vi "Update_Caliper_Overlay_dll.vi"(5 "Analysis_Point_Result":T2[](array[typedef]), 7 "CaliperEntry":T3 {"CaliperType" items=["Distance", "Mid Point", "Perpendicular Projection", "Lines Intersection", "Angle from Horizontal", "Angle from Vertical", "Angle Defined by 3 Points", "Angle Defined by 4 Points", "Bissecting Line", "Mid Line", "Center of Mass", "Area", "Line Fit", "Circle Fit", "Ellipse Fit"]}, 10 "OverlayColor":u32(colorbox)=16711680, 11 "DLL Vision_Image":T1) -> (3 "DLL Vision_Image Out":T1)   [LabVIEW 2019]
uses:
  Caliper/Controls/CaliperDataEntry.ctl
  Caliper/Controls/CaliperType.ctl
  Caliper/Controls/SelectionListEntry.ctl
  Caliper/Controls/SelectionListEntryPointType.ctl
  Caliper/Controls/CaliperResult.ctl
  Analysis/Controls/Analysis_Result_To_Caliper.ctl
  <vilib>/vision/Image Controls.llb/IMAQ Image.ctl
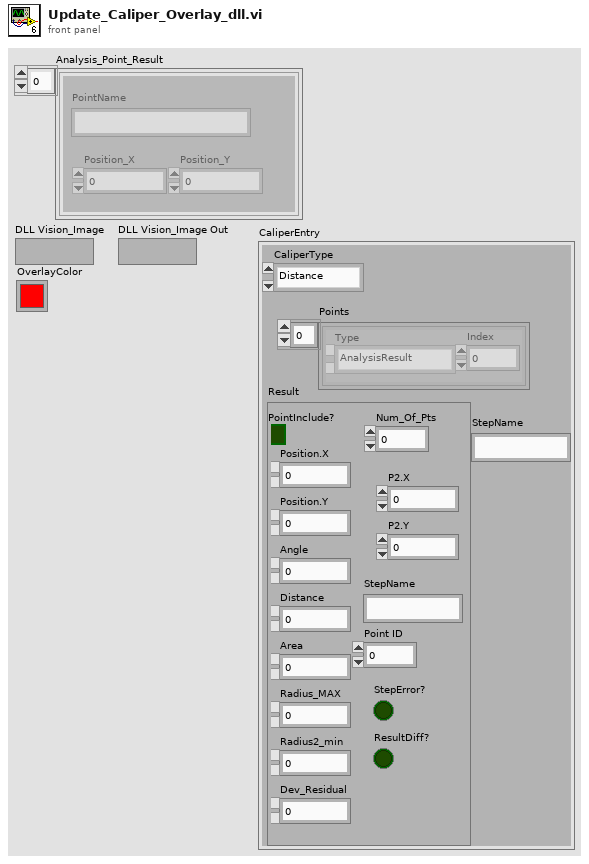
[diagram p1: front panel]
types:
  T1 = typedef "IMAQ Image.ctl" = refnum<image>
  T2 = typedef "Analysis_Result_To_Caliper.ctl" = cluster{"PointName":string, "Position_X":dbl, "Position_Y":dbl}
  T3 = typedef "CaliperDataEntry.ctl" = cluster{"CaliperType":T4, "Points":T5[], "Result":T7, "StepName":string}
  T4 = typedef "CaliperType.ctl" = u32
  T5 = typedef "SelectionListEntry.ctl" = cluster{"Type":T6, "Index":i32}
  T6 = typedef "SelectionListEntryPointType.ctl" = enum16{"AnalysisResult", "CaliperResult"}
  T7 = typedef "CaliperResult.ctl" = cluster{"PointInclude?":bool, "Num_Of_Pts":u8, "Position.X":dbl, "Position.Y":dbl, "Angle":dbl, "Distance":dbl, "Area":dbl, "Radius_MAX":dbl, "Radius2_min":dbl, "Dev_Residual":dbl, "P2.X":dbl, "P2.Y":dbl, "StepName":string, "Point ID":u8, "StepError?":bool, "ResultDiff?":bool}
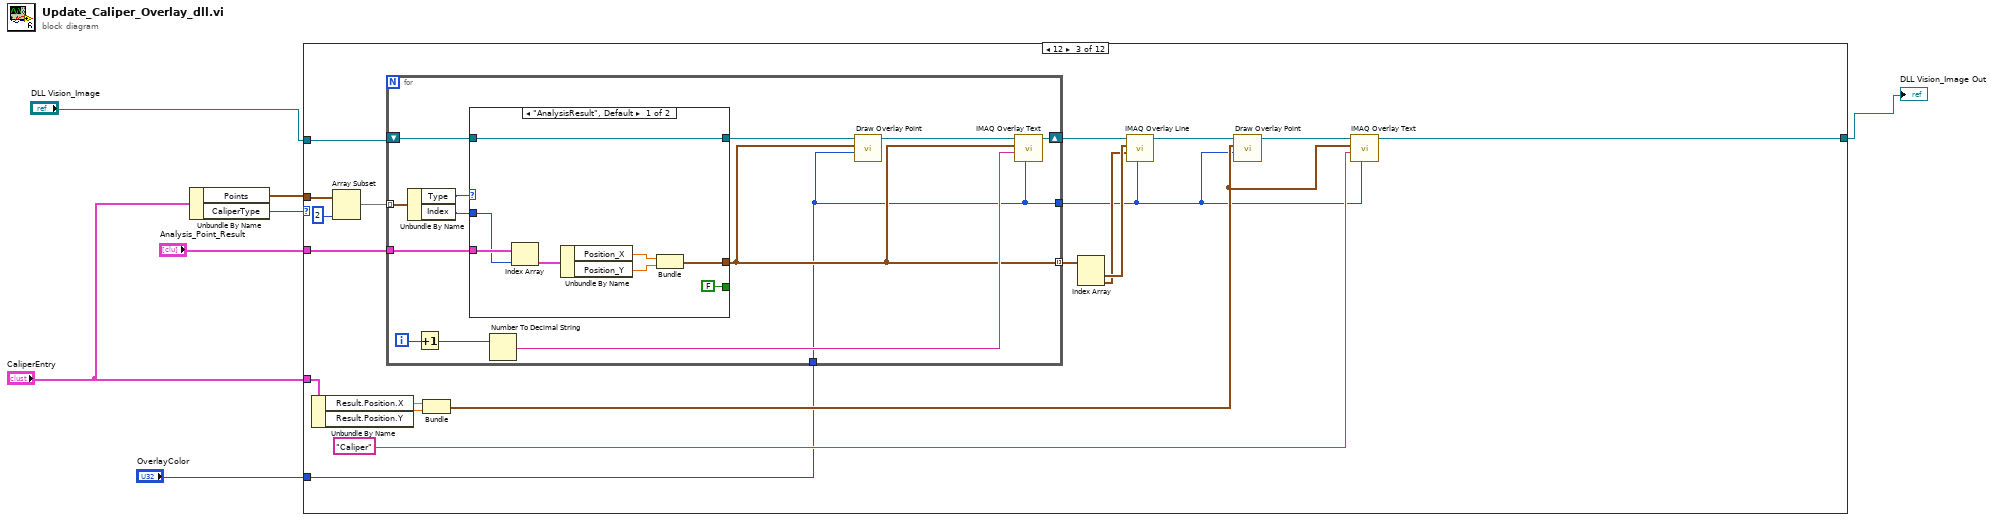
[diagram p0: block diagram]
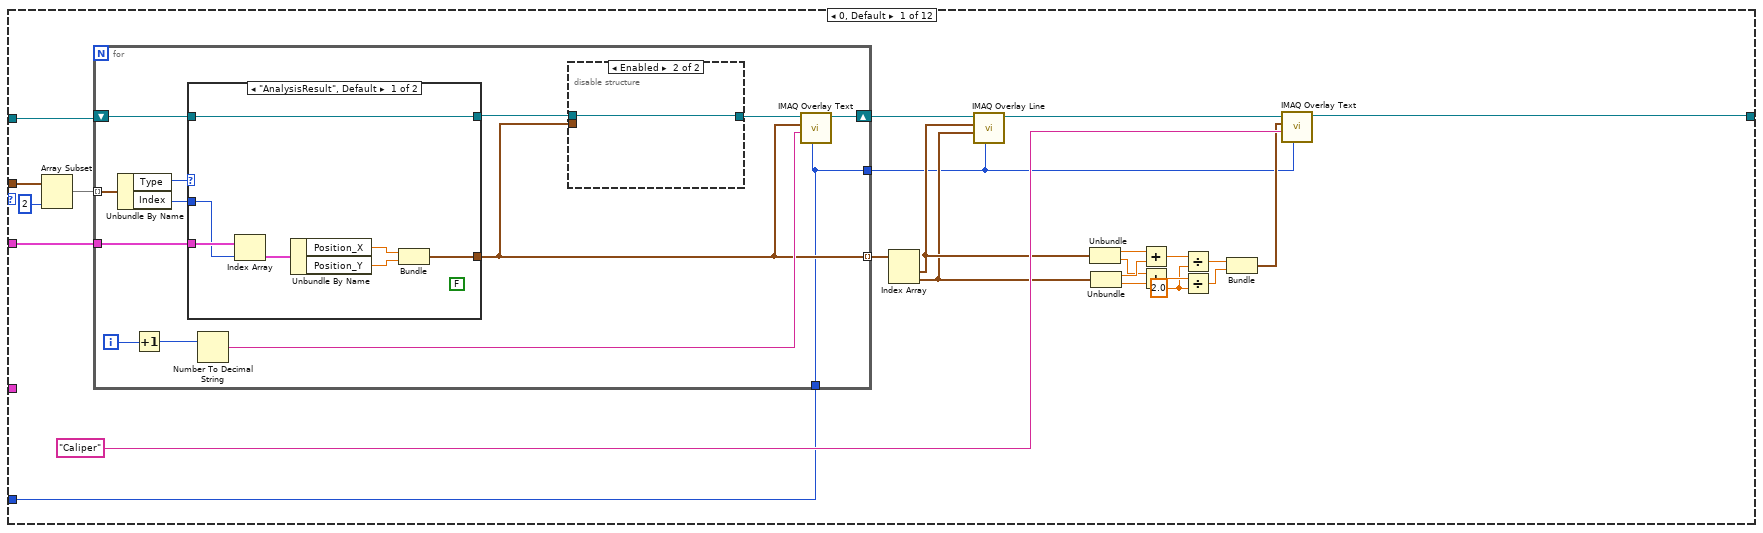
[diagram p2: hidden frame]
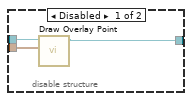
[diagram p3: hidden frame]
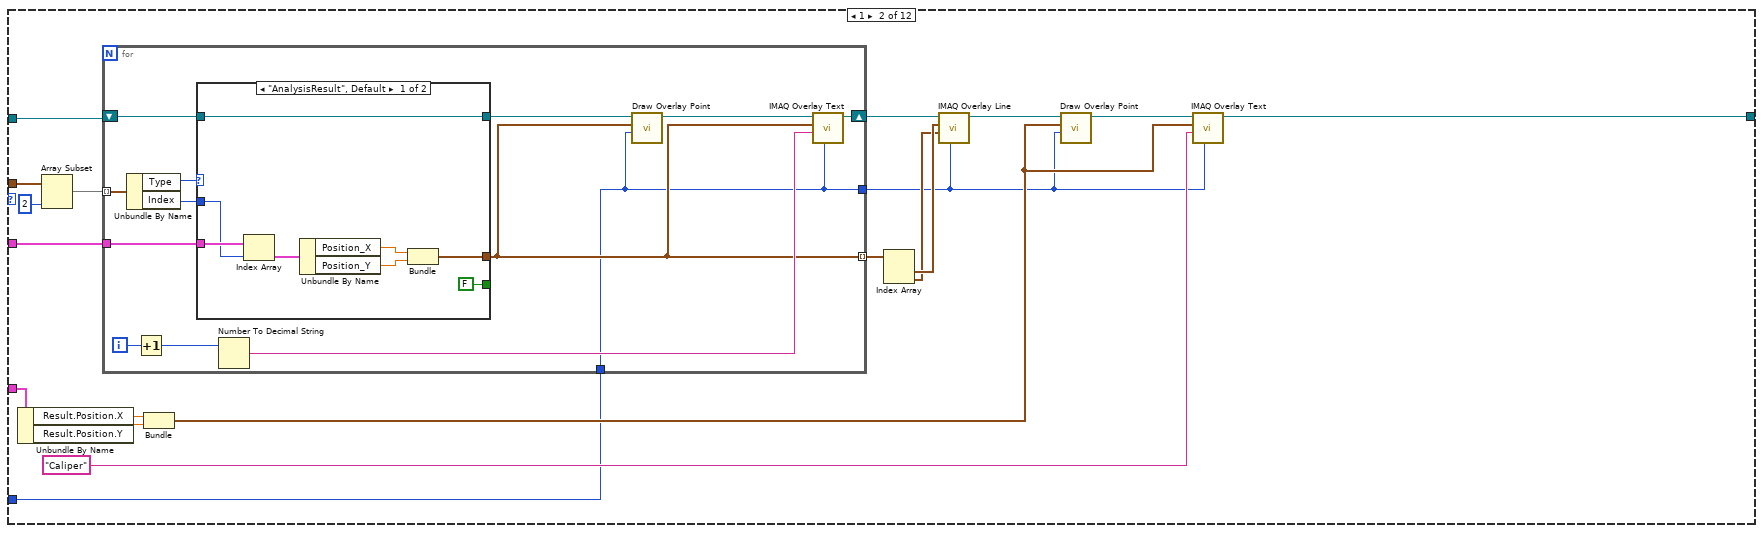
[diagram p5: hidden frame]
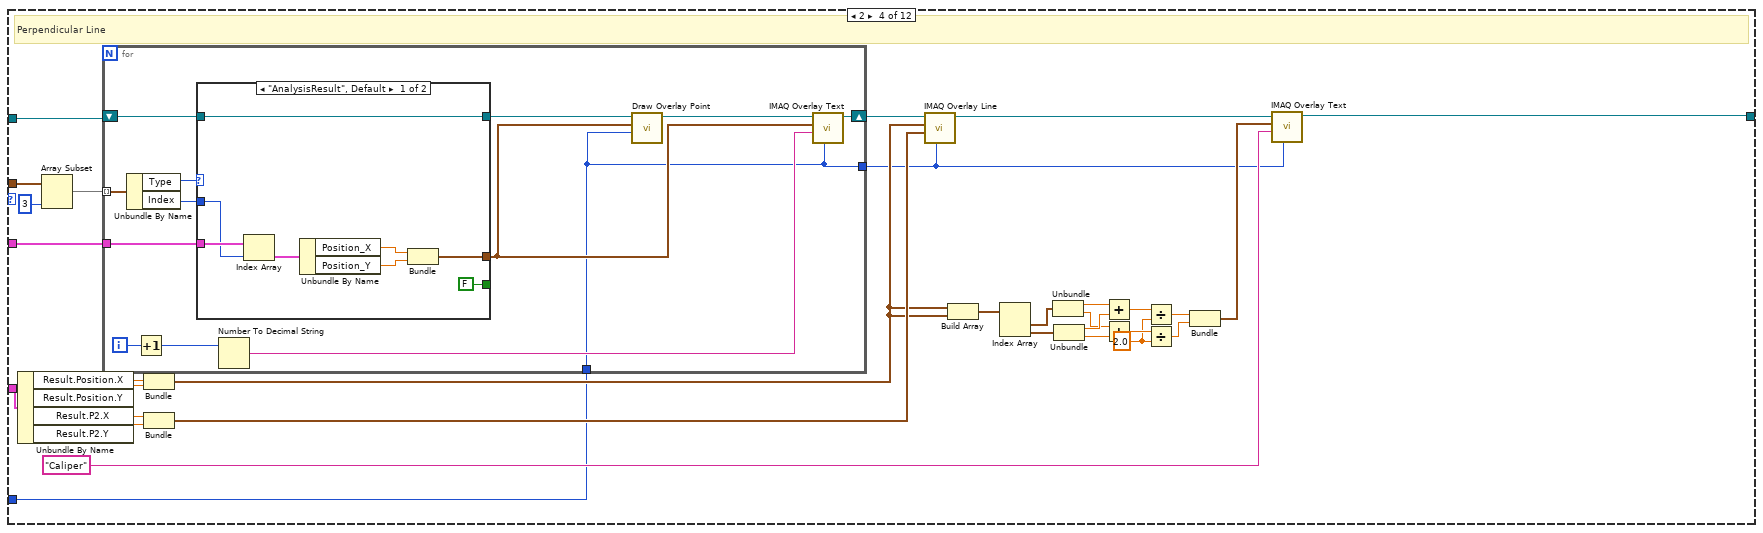
[diagram p8: hidden frame]
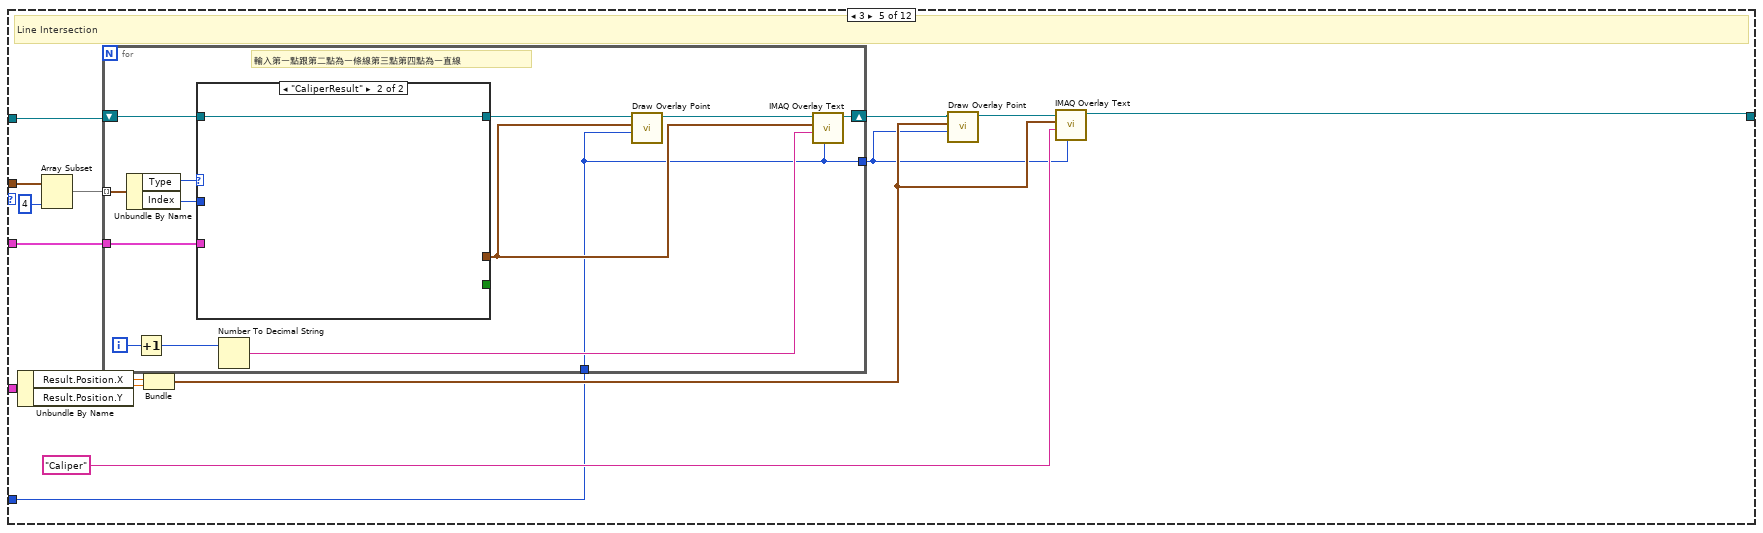
[diagram p10: hidden frame]
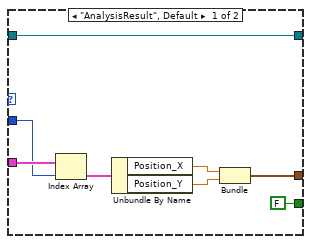
[diagram p11: hidden frame]
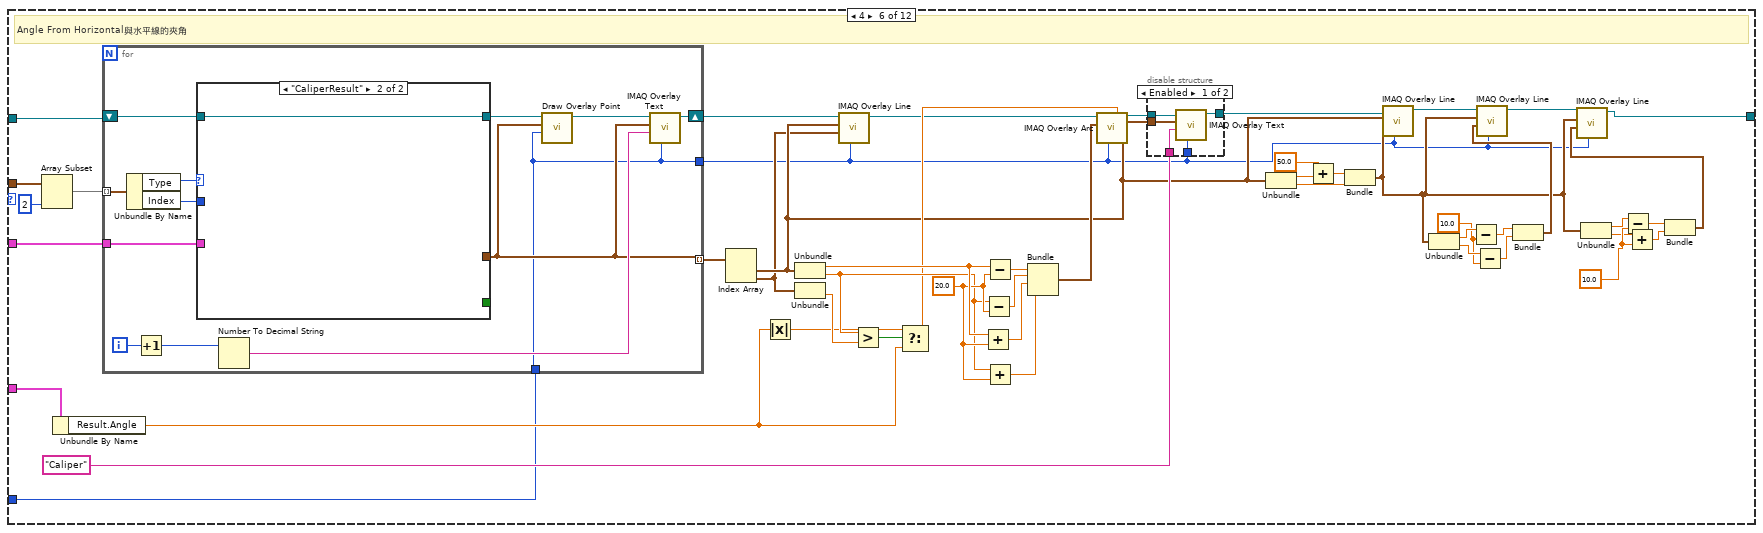
[diagram p12: hidden frame]
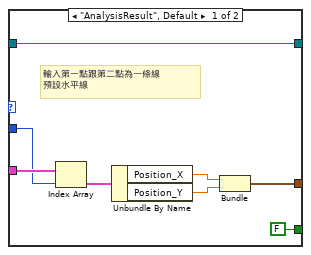
[diagram p14: hidden frame]
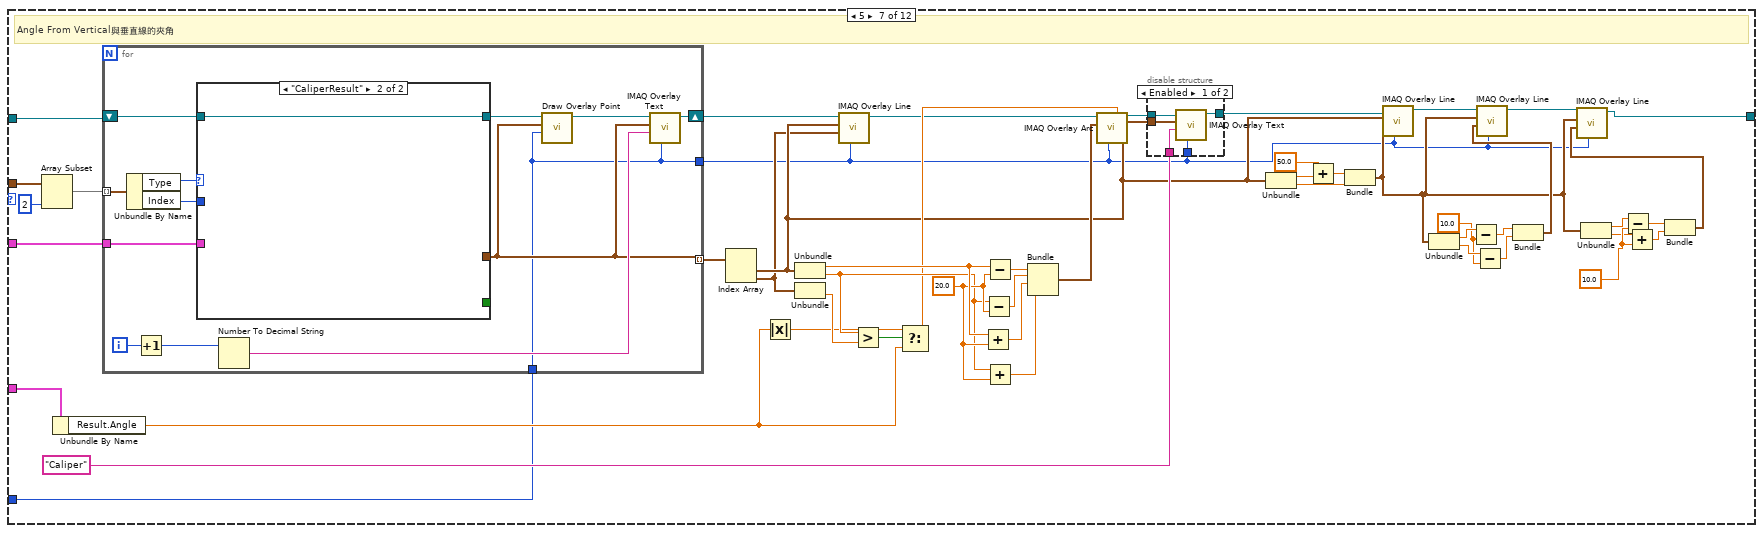
[diagram p15: hidden frame]
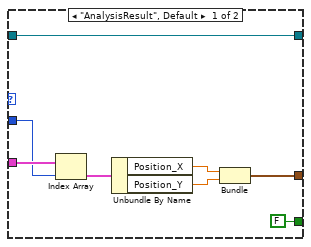
[diagram p17: hidden frame]
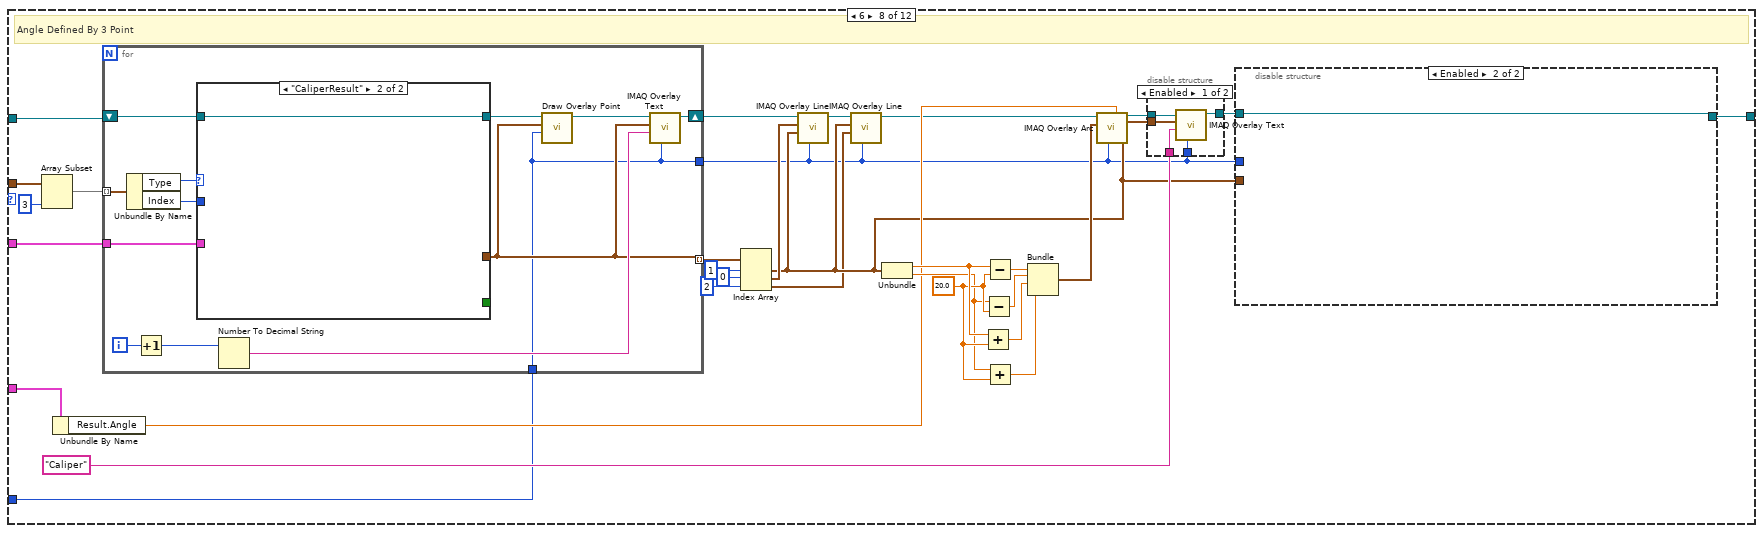
[diagram p18: hidden frame]
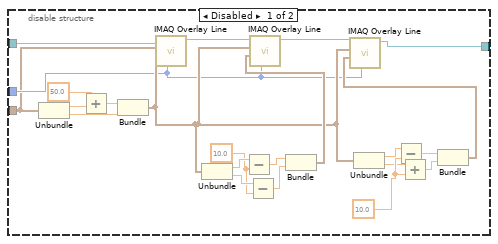
[diagram p19: hidden frame]
diagram:
  n1 = Unbundle By Name("CaliperEntry") -> ("Points"=w5:T5[], "CaliperType"=w4:T4)
  n2 = case shown="12" w4 {
    tunnel: w5 -> [w29 w73 w114 w167 w204 w275 w352 w411 w481 w540 w599 w655]
    tunnel: "Analysis_Point_Result" -> [w28 w72 w113 w166 w203 w274 w351 w410 w480 w539 w598 w654]
    tunnel: "DLL Vision_Image" -> [w27 w63 w104 w162 w201 w272 w349 w408 w478 w537 w596 w652]
    tunnel: [w25 w66 w107 w156 w196 w253 w330 w396 w468 w525 w584 w642] -> w2
    tunnel: "CaliperEntry" -> [_ w71 w112 w165 w202 w273 w350 w409 w479 w538 w597 w653]
    tunnel: "OverlayColor" -> [w8 w58 w99 w139 w192 w230 w307 w384 w466 w507 w565 w624]
    frame 0, Default {
      w16 = 2.0 ("y")
      n3 = Array Subset(array=w29, length=2) -> (w30:T5[])  [unwired: 1 in]
      n4 = for {
        tunnel: w30 -> [w44] mode=indexing
        tunnel: w28 -> [w42]
        shift-right: [w39] -> w26
        shift-left: w27 -> [w40]
        tunnel: [w33] -> w17 mode=indexing
        tunnel: [w32] -> w9
        tunnel: w8 -> [w32]
        i -> [w38]
        n5 = Unbundle By Name(w44) -> ("Type"=w43:T6, "Index"=w41:i32)
        n6 = Increment(x=w38) -> (x+1=w37:i32)
        n7 = case shown="\"AnalysisResult\", Default" w43 {
          tunnel: w42 -> [w55 _]
          tunnel: w41 -> [w54 _]
          tunnel: [w50 _] -> w33
          tunnel: w40 -> [w49 w56]
          tunnel: [w49 w56] -> w35
          frame "AnalysisResult", Default {
            (unwired) FALSE ("StepError?")
            n8 = Index Array(array=w55, index=w54) -> (element=w53:T2)
            n9 = Unbundle By Name(w53) -> ("Position_X"=w52:dbl, "Position_Y"=w51:dbl)
            n10 = Bundle("Position_X"=w52, "Position_Y"=w51) -> (w50:cluster{"Position_X":dbl, "Position_Y":dbl})  [unwired: 1 in]
          }
          frame "CaliperResult" {
          }
        }
        n11 = Number To Decimal String(number=w37) -> (decimal integer string=w36:string)  [unwired: 1 in]
        n12 = disable-structure shown="Enabled" {
          disable-tunnel: w35 -> [w47 w48]
          disable-tunnel: [w46 w48] -> w34
          disable-tunnel: w33 -> [w45 _]
          frame Disabled {
            n13 = call "Draw Overlay Point.vi"("Cluster"=w45, "Refnum in"=w47) -> ("Refnum out"=w46:T1)  [unwired: 9 in]
          }
          frame Enabled {
          }
        }
        n14 = call "IMAQ Overlay Text"("Text Color (black)"=w32, "String"=w36, "Origin"=w33, "Image"=w34) -> ("Image Out"=w39:T1)  [unwired: 6 in, 1 out]
      }
      n15 = Index Array(array=w17) -> (element #1=w11:cluster{"Position_X":dbl, "Position_Y":dbl}, element #2=w10:cluster{"Position_X":dbl, "Position_Y":dbl})  [unwired: 2 in]
      n16 = call "IMAQ Overlay Line"("Color"=w9, "End Point"=w10, "Start Point"=w11, "Image"=w26) -> ("Image Out"=w12:T1)  [unwired: 6 in, 1 out]
      n17 = Unbundle(w11) -> ("Position_X"=w23:dbl, "Position_Y"=w20:dbl)
      n18 = Unbundle(w10) -> ("Position_X"=w21:dbl, "Position_Y"=w22:dbl)
      n19 = Add(x=w23, y=w21) -> (x+y=w19:dbl)
      n20 = Add(x=w20, y=w22) -> (x+y=w18:dbl)
      n21 = Divide(x=w19, y=w16) -> (x/y=w15:dbl)
      n22 = Divide(x=w18, y=w16) -> (x/y=w14:dbl)
      n23 = Bundle(w15, w14) -> (w13:cluster{dbl, dbl})  [unwired: 1 in]
      n24 = call "IMAQ Overlay Text"("Text Color (black)"=w9, "String"="Caliper", "Origin"=w13, "Image"=w12) -> ("Image Out"=w25:T1)  [unwired: 6 in, 1 out]
    }
    frame 1 {
      n25 = Unbundle By Name(w71) -> ("Result.Position.X"=w70:dbl, "Result.Position.Y"=w69:dbl)
      n26 = Array Subset(array=w73, length=2) -> (w74:T5[])  [unwired: 1 in]
      n27 = for {
        tunnel: w74 -> [w88] mode=indexing
        tunnel: w72 -> [w86]
        shift-right: [w81] -> w68
        shift-left: w63 -> [w84]
        tunnel: [w76] -> w57
        tunnel: [w77] -> w61 mode=indexing
        tunnel: w58 -> [w76]
        i -> [w80]
        n28 = Unbundle By Name(w88) -> ("Type"=w87:T6, "Index"=w85:i32)
        n29 = Increment(x=w80) -> (x+1=w78:i32)
        n30 = case shown="\"AnalysisResult\", Default" w87 {
          tunnel: w86 -> [w96 _]
          tunnel: w85 -> [w95 _]
          tunnel: [w91 _] -> w77
          tunnel: [FALSE ("StepError?") _] -> _
          tunnel: w84 -> [w89 w97]
          tunnel: [w89 w97] -> w83
          frame "AnalysisResult", Default {
            n31 = Index Array(array=w96, index=w95) -> (element=w94:T2)
            n32 = Unbundle By Name(w94) -> ("Position_X"=w93:dbl, "Position_Y"=w92:dbl)
            n33 = Bundle("Position_X"=w93, "Position_Y"=w92) -> (w91:cluster{"Position_X":dbl, "Position_Y":dbl})  [unwired: 1 in]
          }
          frame "CaliperResult" {
          }
        }
        n34 = Number To Decimal String(number=w78) -> (decimal integer string=w79:string)  [unwired: 1 in]
        n35 = call "Draw Overlay Point.vi"("Color"=w76, "Cluster"=w77, "Refnum in"=w83) -> ("Refnum out"=w82:T1)  [unwired: 8 in]
        n36 = call "IMAQ Overlay Text"("Text Color (black)"=w76, "String"=w79, "Origin"=w77, "Image"=w82) -> ("Image Out"=w81:T1)  [unwired: 6 in, 1 out]
      }
      n37 = Bundle("Position.X"=w70, "Position.Y"=w69) -> (w65:cluster{"Position.X":dbl, "Position.Y":dbl})  [unwired: 1 in]
      n38 = Index Array(array=w61) -> (element #1=w60:cluster{"Position_X":dbl, "Position_Y":dbl}, element #2=w59:cluster{"Position_X":dbl, "Position_Y":dbl})  [unwired: 2 in]
      n39 = call "IMAQ Overlay Line"("Color"=w57, "End Point"=w59, "Start Point"=w60, "Image"=w68) -> ("Image Out"=w62:T1)  [unwired: 6 in, 1 out]
      n40 = call "Draw Overlay Point.vi"("Color"=w57, "Cluster"=w65, "Refnum in"=w62) -> ("Refnum out"=w67:T1)  [unwired: 8 in]
      n41 = call "IMAQ Overlay Text"("Text Color (black)"=w57, "String"="Caliper", "Origin"=w65, "Image"=w67) -> ("Image Out"=w66:T1)  [unwired: 6 in, 1 out]
    }
    frame 12 {
      n42 = Unbundle By Name(w112) -> ("Result.Position.X"=w111:dbl, "Result.Position.Y"=w110:dbl)
      n43 = Array Subset(array=w114, length=2) -> (w115:T5[])  [unwired: 1 in]
      n44 = for {
        tunnel: w115 -> [w129] mode=indexing
        tunnel: w113 -> [w127]
        shift-right: [w122] -> w109
        shift-left: w104 -> [w125]
        tunnel: [w117] -> w98
        tunnel: [w118] -> w102 mode=indexing
        tunnel: w99 -> [w117]
        i -> [w121]
        n45 = Unbundle By Name(w129) -> ("Type"=w128:T6, "Index"=w126:i32)
        n46 = Increment(x=w121) -> (x+1=w119:i32)
        n47 = case shown="\"AnalysisResult\", Default" w128 {
          tunnel: w127 -> [w137 _]
          tunnel: w126 -> [w136 _]
          tunnel: [w132 _] -> w118
          tunnel: [FALSE ("StepError?") _] -> _
          tunnel: w125 -> [w130 w138]
          tunnel: [w130 w138] -> w124
          frame "AnalysisResult", Default {
            n48 = Index Array(array=w137, index=w136) -> (element=w135:T2)
            n49 = Unbundle By Name(w135) -> ("Position_X"=w134:dbl, "Position_Y"=w133:dbl)
            n50 = Bundle("Position_X"=w134, "Position_Y"=w133) -> (w132:cluster{"Position_X":dbl, "Position_Y":dbl})  [unwired: 1 in]
          }
          frame "CaliperResult" {
          }
        }
        n51 = Number To Decimal String(number=w119) -> (decimal integer string=w120:string)  [unwired: 1 in]
        n52 = call "Draw Overlay Point.vi"("Color"=w117, "Cluster"=w118, "Refnum in"=w124) -> ("Refnum out"=w123:T1)  [unwired: 8 in]
        n53 = call "IMAQ Overlay Text"("Text Color (black)"=w117, "String"=w120, "Origin"=w118, "Image"=w123) -> ("Image Out"=w122:T1)  [unwired: 6 in, 1 out]
      }
      n54 = Bundle("Position.X"=w111, "Position.Y"=w110) -> (w106:cluster{"Position.X":dbl, "Position.Y":dbl})  [unwired: 1 in]
      n55 = Index Array(array=w102) -> (element #1=w101:cluster{"Position_X":dbl, "Position_Y":dbl}, element #2=w100:cluster{"Position_X":dbl, "Position_Y":dbl})  [unwired: 2 in]
      n56 = call "IMAQ Overlay Line"("Color"=w98, "End Point"=w100, "Start Point"=w101, "Image"=w109) -> ("Image Out"=w103:T1)  [unwired: 6 in, 1 out]
      n57 = call "Draw Overlay Point.vi"("Color"=w98, "Cluster"=w106, "Refnum in"=w103) -> ("Refnum out"=w108:T1)  [unwired: 8 in]
      n58 = call "IMAQ Overlay Text"("Text Color (black)"=w98, "String"="Caliper", "Origin"=w106, "Image"=w108) -> ("Image Out"=w107:T1)  [unwired: 6 in, 1 out]
    }
    frame 2 {
      w146 = 2.0 ("y")
      # "Perpendicular Line"
      n59 = Unbundle By Name(w165) -> ("Result.Position.X"=w161:dbl, "Result.Position.Y"=w160:dbl, "Result.P2.X"=w164:dbl, "Result.P2.Y"=w163:dbl)
      n60 = Array Subset(array=w167, length=3) -> (w168:T5[])  [unwired: 1 in]
      n61 = for {
        tunnel: w168 -> [w182] mode=indexing
        tunnel: w166 -> [w180]
        shift-right: [w175] -> w159
        shift-left: w162 -> [w178]
        tunnel: [w170] -> w140
        tunnel: w139 -> [w170]
        i -> [w173]
        n62 = Unbundle By Name(w182) -> ("Type"=w181:T6, "Index"=w179:i32)
        n63 = Increment(x=w173) -> (x+1=w171:i32)
        n64 = case shown="\"AnalysisResult\", Default" w181 {
          tunnel: w180 -> [w190 _]
          tunnel: w179 -> [w189 _]
          tunnel: [w185 _] -> w174
          tunnel: [FALSE ("StepError?") _] -> _
          tunnel: w178 -> [w183 w191]
          tunnel: [w183 w191] -> w177
          frame "AnalysisResult", Default {
            n65 = Index Array(array=w190, index=w189) -> (element=w188:T2)
            n66 = Unbundle By Name(w188) -> ("Position_X"=w187:dbl, "Position_Y"=w186:dbl)
            n67 = Bundle("Position_X"=w187, "Position_Y"=w186) -> (w185:cluster{"Position_X":dbl, "Position_Y":dbl})  [unwired: 1 in]
          }
          frame "CaliperResult" {
          }
        }
        n68 = Number To Decimal String(number=w171) -> (decimal integer string=w172:string)  [unwired: 1 in]
        n69 = call "Draw Overlay Point.vi"("Color"=w170, "Cluster"=w174, "Refnum in"=w177) -> ("Refnum out"=w176:T1)  [unwired: 8 in]
        n70 = call "IMAQ Overlay Text"("Text Color (black)"=w170, "String"=w172, "Origin"=w174, "Image"=w176) -> ("Image Out"=w175:T1)  [unwired: 6 in, 1 out]
      }
      n71 = Bundle("Position.X"=w161, "Position.Y"=w160) -> (w155:cluster{"Position.X":dbl, "Position.Y":dbl})  [unwired: 1 in]
      n72 = Bundle("P2.X"=w164, "P2.Y"=w163) -> (w158:cluster{"P2.X":dbl, "P2.Y":dbl})  [unwired: 1 in]
      n73 = call "IMAQ Overlay Line"("Color"=w140, "End Point"=w158, "Start Point"=w155, "Image"=w159) -> ("Image Out"=w157:T1)  [unwired: 6 in, 1 out]
      n74 = Build Array(w155, w155) -> (w143:cluster{"Position.X":dbl, "Position.Y":dbl}[])
      n75 = Index Array(array=w143) -> (element #1=w154:cluster{"Position.X":dbl, "Position.Y":dbl}, element #2=w147:cluster{"Position.X":dbl, "Position.Y":dbl})  [unwired: 2 in]
      n76 = Unbundle(w154) -> ("Position.X"=w153:dbl, "Position.Y"=w150:dbl)
      n77 = Unbundle(w147) -> ("Position.X"=w151:dbl, "Position.Y"=w152:dbl)
      n78 = Add(x=w153, y=w151) -> (x+y=w149:dbl)
      n79 = Add(x=w150, y=w152) -> (x+y=w148:dbl)
      n80 = Divide(x=w149, y=w146) -> (x/y=w145:dbl)
      n81 = Divide(x=w148, y=w146) -> (x/y=w144:dbl)
      n82 = Bundle(w145, w144) -> (w142:cluster{dbl, dbl})  [unwired: 1 in]
      n83 = call "IMAQ Overlay Text"("Text Color (black)"=w140, "String"="Caliper", "Origin"=w142, "Image"=w157) -> ("Image Out"=w156:T1)  [unwired: 6 in, 1 out]
    }
    frame 3 {
      # "Line Intersection"
      n84 = Unbundle By Name(w202) -> ("Result.Position.X"=w200:dbl, "Result.Position.Y"=w199:dbl)
      n85 = Array Subset(array=w204, length=4) -> (w205:T5[])  [unwired: 1 in]
      n86 = for {
        tunnel: w205 -> [w219] mode=indexing
        tunnel: w203 -> [w217]
        shift-right: [w212] -> w198
        shift-left: w201 -> [w215]
        tunnel: [w207] -> w193
        tunnel: w192 -> [w207]
        i -> [w210]
        # "輸入第一點跟第二點為一條線第三點第四點為一直線"
        n87 = Unbundle By Name(w219) -> ("Type"=w218:T6, "Index"=w216:i32)
        n88 = Increment(x=w210) -> (x+1=w208:i32)
        n89 = case shown="\"CaliperResult\"" w218 {
          tunnel: w217 -> [w227 _]
          tunnel: w216 -> [w226 _]
          tunnel: [w222 _] -> w211
          tunnel: [FALSE ("StepError?") _] -> _
          tunnel: w215 -> [w220 w228]
          tunnel: [w220 w228] -> w214
          frame "AnalysisResult", Default {
            n90 = Index Array(array=w227, index=w226) -> (element=w225:T2)
            n91 = Unbundle By Name(w225) -> ("Position_X"=w224:dbl, "Position_Y"=w223:dbl)
            n92 = Bundle("Position_X"=w224, "Position_Y"=w223) -> (w222:cluster{"Position_X":dbl, "Position_Y":dbl})  [unwired: 1 in]
          }
          frame "CaliperResult" {
          }
        }
        n93 = Number To Decimal String(number=w208) -> (decimal integer string=w209:string)  [unwired: 1 in]
        n94 = call "Draw Overlay Point.vi"("Color"=w207, "Cluster"=w211, "Refnum in"=w214) -> ("Refnum out"=w213:T1)  [unwired: 8 in]
        n95 = call "IMAQ Overlay Text"("Text Color (black)"=w207, "String"=w209, "Origin"=w211, "Image"=w213) -> ("Image Out"=w212:T1)  [unwired: 6 in, 1 out]
      }
      n96 = Bundle("Position.X"=w200, "Position.Y"=w199) -> (w195:cluster{"Position.X":dbl, "Position.Y":dbl})  [unwired: 1 in]
      n97 = call "Draw Overlay Point.vi"("Color"=w193, "Cluster"=w195, "Refnum in"=w198) -> ("Refnum out"=w197:T1)  [unwired: 8 in]
      n98 = call "IMAQ Overlay Text"("Text Color (black)"=w193, "String"="Caliper", "Origin"=w195, "Image"=w197) -> ("Image Out"=w196:T1)  [unwired: 6 in, 1 out]
    }
    frame 4 {
      w241 = 10.0 ("x")
      w243 = 10.0 ("x")
      w266 = 20.0
      # "Angle From Horizontal與水平線的夾角"
      n99 = Array Subset(array=w275, length=2) -> (w276:T5[])  [unwired: 1 in]
      n100 = Unbundle By Name(w273) -> ("Result.Angle"=w235:dbl)
      n101 = for {
        tunnel: w276 -> [w296] mode=indexing
        tunnel: w274 -> [w294]
        shift-right: [w289] -> w270
        shift-left: w272 -> [w292]
        tunnel: [w284] -> w229
        tunnel: [w285] -> w268 mode=indexing
        tunnel: w230 -> [w284]
        i -> [w288]
        n102 = Unbundle By Name(w296) -> ("Type"=w295:T6, "Index"=w293:i32)
        n103 = Increment(x=w288) -> (x+1=w286:i32)
        n104 = case shown="\"CaliperResult\"" w295 {
          tunnel: w294 -> [w304 _]
          tunnel: w293 -> [w303 _]
          tunnel: [w299 _] -> w285
          tunnel: [FALSE ("StepError?") _] -> _
          tunnel: w292 -> [w297 w305]
          tunnel: [w297 w305] -> w291
          frame "AnalysisResult", Default {
            # "輸入第一點跟第二點為一條線\n預設水平線"
            n105 = Index Array(array=w304, index=w303) -> (element=w302:T2)
            n106 = Unbundle By Name(w302) -> ("Position_X"=w301:dbl, "Position_Y"=w300:dbl)
            n107 = Bundle("Position_X"=w301, "Position_Y"=w300) -> (w299:cluster{"Position_X":dbl, "Position_Y":dbl})  [unwired: 1 in]
          }
          frame "CaliperResult" {
          }
        }
        n108 = Number To Decimal String(number=w286) -> (decimal integer string=w287:string)  [unwired: 1 in]
        n109 = call "Draw Overlay Point.vi"("Color"=w284, "Cluster"=w285, "Refnum in"=w291) -> ("Refnum out"=w290:T1)  [unwired: 8 in]
        n110 = call "IMAQ Overlay Text"("Text Color (black)"=w284, "String"=w287, "Origin"=w285, "Image"=w290) -> ("Image Out"=w289:T1)  [unwired: 6 in, 1 out]
      }
      n111 = Index Array(array=w268) -> (element #1=w232:cluster{"Position_X":dbl, "Position_Y":dbl}, element #2=w231:cluster{"Position_X":dbl, "Position_Y":dbl})  [unwired: 2 in]
      n112 = Absolute Value(x=w235) -> (abs(x)=w236:dbl)
      n113 = Unbundle(w232) -> ("Position_X"=w267:dbl, "Position_Y"=w239:dbl)
      n114 = Unbundle(w231) -> ("Position_Y"=w238:dbl)  [unwired: 1 out]
      n115 = call "IMAQ Overlay Line"("Color"=w229, "End Point"=w231, "Start Point"=w232, "Image"=w270) -> ("Image Out"=w233:T1)  [unwired: 6 in, 1 out]
      n116 = Greater?(x=w239, y=w238) -> (0:w237:bool)
      n117 = Select(t=w236, s=w237, f=w235) -> (s? t:f=w234:dbl)
      n118 = Add(x=w267, y=w266) -> (x+y=w263:dbl)
      n119 = Subtract(x=w239, y=w266) -> (x-y=w264:dbl)
      n120 = Subtract(x=w267, y=w266) -> (x-y=w265:dbl)
      n121 = Add(x=w239, y=w266) -> (x+y=w262:dbl)
      n122 = Bundle(w265, w264, w263, w262) -> (w261:cluster{dbl, dbl, dbl, dbl})  [unwired: 1 in]
      n123 = call "IMAQ Overlay Arc"("End Angle (degrees)"=w234, "Color"=w229, "Bounding Rectangle"=w261, "Image"=w233) -> ("Image Out"=w269:T1)  [unwired: 6 in, 1 out]
      n124 = disable-structure shown="Enabled" {
        disable-tunnel: [w282 w283] -> w260
        disable-tunnel: "Caliper" -> [w281 _]
        disable-tunnel: w229 -> [w280 _]
        disable-tunnel: w269 -> [w279 w283]
        disable-tunnel: w232 -> [w278 _]
        frame Enabled {
          n125 = call "IMAQ Overlay Text"("Text Color (black)"=w280, "String"=w281, "Origin"=w278, "Image"=w279) -> ("Image Out"=w282:T1)  [unwired: 6 in, 1 out]
        }
        frame Disabled {
        }
      }
      n126 = Unbundle(w232) -> ("Position_X"=w259:dbl, "Position_Y"=w256:dbl)
      n127 = Add(x=50.0, y=w259) -> (x+y=w257:dbl)
      n128 = Bundle(w257, "Position_Y"=w256) -> (w246:cluster{dbl, "Position_Y":dbl})  [unwired: 1 in]
      n129 = call "IMAQ Overlay Line"("Color"=w229, "End Point"=w246, "Start Point"=w232, "Image"=w260) -> ("Image Out"=w255:T1)  [unwired: 6 in, 1 out]
      n130 = Unbundle(w246) -> (w245:dbl, "Position_Y"=w244:dbl)
      n131 = Subtract(x=w245, y=w243) -> (x-y=w252:dbl)
      n132 = Subtract(x=w244, y=w243) -> (x-y=w251:dbl)
      n133 = Bundle(w252, w251) -> (w250:cluster{dbl, dbl})  [unwired: 1 in]
      n134 = call "IMAQ Overlay Line"("Color"=w229, "End Point"=w250, "Start Point"=w246, "Image"=w255) -> ("Image Out"=w254:T1)  [unwired: 6 in, 1 out]
      n135 = Unbundle(w246) -> (w242:dbl, "Position_Y"=w240:dbl)
      n136 = Subtract(x=w242, y=w241) -> (x-y=w248:dbl)
      n137 = Add(x=w240, y=w241) -> (x+y=w249:dbl)
      n138 = Bundle(w248, w249) -> (w247:cluster{dbl, dbl})  [unwired: 1 in]
      n139 = call "IMAQ Overlay Line"("Color"=w229, "End Point"=w247, "Start Point"=w246, "Image"=w254) -> ("Image Out"=w253:T1)  [unwired: 6 in, 1 out]
    }
    frame 5 {
      w318 = 10.0 ("x")
      w320 = 10.0 ("x")
      w343 = 20.0
      # "Angle From Vertical與垂直線的夾角"
      n140 = Array Subset(array=w352, length=2) -> (w353:T5[])  [unwired: 1 in]
      n141 = Unbundle By Name(w350) -> ("Result.Angle"=w312:dbl)
      n142 = for {
        tunnel: w353 -> [w373] mode=indexing
        tunnel: w351 -> [w371]
        shift-right: [w366] -> w347
        shift-left: w349 -> [w369]
        tunnel: [w361] -> w306
        tunnel: [w362] -> w345 mode=indexing
        tunnel: w307 -> [w361]
        i -> [w365]
        n143 = Unbundle By Name(w373) -> ("Type"=w372:T6, "Index"=w370:i32)
        n144 = Increment(x=w365) -> (x+1=w363:i32)
        n145 = case shown="\"CaliperResult\"" w372 {
          tunnel: w371 -> [w381 _]
          tunnel: w370 -> [w380 _]
          tunnel: [w376 _] -> w362
          tunnel: [FALSE ("StepError?") _] -> _
          tunnel: w369 -> [w374 w382]
          tunnel: [w374 w382] -> w368
          frame "AnalysisResult", Default {
            n146 = Index Array(array=w381, index=w380) -> (element=w379:T2)
            n147 = Unbundle By Name(w379) -> ("Position_X"=w378:dbl, "Position_Y"=w377:dbl)
            n148 = Bundle("Position_X"=w378, "Position_Y"=w377) -> (w376:cluster{"Position_X":dbl, "Position_Y":dbl})  [unwired: 1 in]
          }
          frame "CaliperResult" {
          }
        }
        n149 = Number To Decimal String(number=w363) -> (decimal integer string=w364:string)  [unwired: 1 in]
        n150 = call "Draw Overlay Point.vi"("Color"=w361, "Cluster"=w362, "Refnum in"=w368) -> ("Refnum out"=w367:T1)  [unwired: 8 in]
        n151 = call "IMAQ Overlay Text"("Text Color (black)"=w361, "String"=w364, "Origin"=w362, "Image"=w367) -> ("Image Out"=w366:T1)  [unwired: 6 in, 1 out]
      }
      n152 = Index Array(array=w345) -> (element #1=w309:cluster{"Position_X":dbl, "Position_Y":dbl}, element #2=w308:cluster{"Position_X":dbl, "Position_Y":dbl})  [unwired: 2 in]
      n153 = Absolute Value(x=w312) -> (abs(x)=w313:dbl)
      n154 = Unbundle(w309) -> ("Position_X"=w344:dbl, "Position_Y"=w316:dbl)
      n155 = Unbundle(w308) -> ("Position_Y"=w315:dbl)  [unwired: 1 out]
      n156 = call "IMAQ Overlay Line"("Color"=w306, "End Point"=w308, "Start Point"=w309, "Image"=w347) -> ("Image Out"=w310:T1)  [unwired: 6 in, 1 out]
      n157 = Greater?(x=w316, y=w315) -> (0:w314:bool)
      n158 = Select(t=w313, s=w314, f=w312) -> (s? t:f=w311:dbl)
      n159 = Add(x=w344, y=w343) -> (x+y=w340:dbl)
      n160 = Subtract(x=w316, y=w343) -> (x-y=w341:dbl)
      n161 = Subtract(x=w344, y=w343) -> (x-y=w342:dbl)
      n162 = Add(x=w316, y=w343) -> (x+y=w339:dbl)
      n163 = Bundle(w342, w341, w340, w339) -> (w338:cluster{dbl, dbl, dbl, dbl})  [unwired: 1 in]
      n164 = call "IMAQ Overlay Arc"("End Angle (degrees)"=w311, "Color"=w306, "Bounding Rectangle"=w338, "Image"=w310) -> ("Image Out"=w346:T1)  [unwired: 6 in, 1 out]
      n165 = disable-structure shown="Enabled" {
        disable-tunnel: [w359 w360] -> w337
        disable-tunnel: "Caliper" -> [w358 _]
        disable-tunnel: w306 -> [w357 _]
        disable-tunnel: w346 -> [w356 w360]
        disable-tunnel: w309 -> [w355 _]
        frame Enabled {
          n166 = call "IMAQ Overlay Text"("Text Color (black)"=w357, "String"=w358, "Origin"=w355, "Image"=w356) -> ("Image Out"=w359:T1)  [unwired: 6 in, 1 out]
        }
        frame Disabled {
        }
      }
      n167 = Unbundle(w309) -> ("Position_X"=w336:dbl, "Position_Y"=w333:dbl)
      n168 = Add(x=50.0, y=w336) -> (x+y=w334:dbl)
      n169 = Bundle(w334, "Position_Y"=w333) -> (w323:cluster{dbl, "Position_Y":dbl})  [unwired: 1 in]
      n170 = call "IMAQ Overlay Line"("Color"=w306, "End Point"=w323, "Start Point"=w309, "Image"=w337) -> ("Image Out"=w332:T1)  [unwired: 6 in, 1 out]
      n171 = Unbundle(w323) -> (w322:dbl, "Position_Y"=w321:dbl)
      n172 = Subtract(x=w322, y=w320) -> (x-y=w329:dbl)
      n173 = Subtract(x=w321, y=w320) -> (x-y=w328:dbl)
      n174 = Bundle(w329, w328) -> (w327:cluster{dbl, dbl})  [unwired: 1 in]
      n175 = call "IMAQ Overlay Line"("Color"=w306, "End Point"=w327, "Start Point"=w323, "Image"=w332) -> ("Image Out"=w331:T1)  [unwired: 6 in, 1 out]
      n176 = Unbundle(w323) -> (w319:dbl, "Position_Y"=w317:dbl)
      n177 = Subtract(x=w319, y=w318) -> (x-y=w325:dbl)
      n178 = Add(x=w317, y=w318) -> (x+y=w326:dbl)
      n179 = Bundle(w325, w326) -> (w324:cluster{dbl, dbl})  [unwired: 1 in]
      n180 = call "IMAQ Overlay Line"("Color"=w306, "End Point"=w324, "Start Point"=w323, "Image"=w331) -> ("Image Out"=w330:T1)  [unwired: 6 in, 1 out]
    }
    frame 6 {
      w403 = 20.0
      # "Angle Defined By 3 Point"
      n181 = Array Subset(array=w411, length=3) -> (w412:T5[])  [unwired: 1 in]
      n182 = Unbundle By Name(w409) -> ("Result.Angle"=w393:dbl)
      n183 = for {
        tunnel: w412 -> [w456] mode=indexing
        tunnel: w410 -> [w454]
        shift-right: [w449] -> w394
        shift-left: w408 -> [w452]
        tunnel: [w444] -> w383
        tunnel: [w445] -> w405 mode=indexing
        tunnel: w384 -> [w444]
        i -> [w448]
        n184 = Unbundle By Name(w456) -> ("Type"=w455:T6, "Index"=w453:i32)
        n185 = Increment(x=w448) -> (x+1=w446:i32)
        n186 = case shown="\"CaliperResult\"" w455 {
          tunnel: w454 -> [w464 _]
          tunnel: w453 -> [w463 _]
          tunnel: [w459 _] -> w445
          tunnel: [FALSE ("StepError?") _] -> _
          tunnel: w452 -> [w457 w465]
          tunnel: [w457 w465] -> w451
          frame "AnalysisResult", Default {
            n187 = Index Array(array=w464, index=w463) -> (element=w462:T2)
            n188 = Unbundle By Name(w462) -> ("Position_X"=w461:dbl, "Position_Y"=w460:dbl)
            n189 = Bundle("Position_X"=w461, "Position_Y"=w460) -> (w459:cluster{"Position_X":dbl, "Position_Y":dbl})  [unwired: 1 in]
          }
          frame "CaliperResult" {
          }
        }
        n190 = Number To Decimal String(number=w446) -> (decimal integer string=w447:string)  [unwired: 1 in]
        n191 = call "Draw Overlay Point.vi"("Color"=w444, "Cluster"=w445, "Refnum in"=w451) -> ("Refnum out"=w450:T1)  [unwired: 8 in]
        n192 = call "IMAQ Overlay Text"("Text Color (black)"=w444, "String"=w447, "Origin"=w445, "Image"=w450) -> ("Image Out"=w449:T1)  [unwired: 6 in, 1 out]
      }
      n193 = Index Array(array=w405, index #1=1 ("index"), index #2=0 ("index"), index #3=2 ("index")) -> (element #1=w386:cluster{"Position_X":dbl, "Position_Y":dbl}, element #2=w388:cluster{"Position_X":dbl, "Position_Y":dbl}, element #3=w385:cluster{"Position_X":dbl, "Position_Y":dbl})
      n194 = call "IMAQ Overlay Line"("Color"=w383, "End Point"=w386, "Start Point"=w388, "Image"=w394) -> ("Image Out"=w391:T1)  [unwired: 6 in, 1 out]
      n195 = call "IMAQ Overlay Line"("Color"=w383, "End Point"=w385, "Start Point"=w386, "Image"=w391) -> ("Image Out"=w387:T1)  [unwired: 6 in, 1 out]
      n196 = Unbundle(w386) -> ("Position_X"=w404:dbl, "Position_Y"=w395:dbl)
      n197 = Add(x=w404, y=w403) -> (x+y=w400:dbl)
      n198 = Subtract(x=w395, y=w403) -> (x-y=w401:dbl)
      n199 = Subtract(x=w404, y=w403) -> (x-y=w402:dbl)
      n200 = Add(x=w395, y=w403) -> (x+y=w399:dbl)
      n201 = Bundle(w402, w401, w400, w399) -> (w398:cluster{dbl, dbl, dbl, dbl})  [unwired: 1 in]
      n202 = call "IMAQ Overlay Arc"("End Angle (degrees)"=w393, "Color"=w383, "Bounding Rectangle"=w398, "Image"=w387) -> ("Image Out"=w406:T1)  [unwired: 6 in, 1 out]
      n203 = disable-structure shown="Enabled" {
        disable-tunnel: [w442 w443] -> w397
        disable-tunnel: "Caliper" -> [w441 _]
        disable-tunnel: w383 -> [w440 _]
        disable-tunnel: w406 -> [w439 w443]
        disable-tunnel: w386 -> [w438 _]
        frame Enabled {
          n204 = call "IMAQ Overlay Text"("Text Color (black)"=w440, "String"=w441, "Origin"=w438, "Image"=w439) -> ("Image Out"=w442:T1)  [unwired: 6 in, 1 out]
        }
        frame Disabled {
        }
      }
      n205 = disable-structure shown="Enabled" {
        disable-tunnel: w397 -> [w436 w437]
        disable-tunnel: [w429 w437] -> w396
        disable-tunnel: w383 -> [w415 _]
        disable-tunnel: w386 -> [w414 _]
        frame Disabled {
          w417 = 10.0 ("x")
          w419 = 10.0 ("x")
          n206 = Unbundle(w414) -> ("Position_X"=w435:dbl, "Position_Y"=w432:dbl)
          n207 = Add(x=50.0, y=w435) -> (x+y=w433:dbl)
          n208 = Bundle(w433, "Position_Y"=w432) -> (w422:cluster{dbl, "Position_Y":dbl})  [unwired: 1 in]
          n209 = call "IMAQ Overlay Line"("Color"=w415, "End Point"=w422, "Start Point"=w414, "Image"=w436) -> ("Image Out"=w431:T1)  [unwired: 6 in, 1 out]
          n210 = Unbundle(w422) -> (w421:dbl, "Position_Y"=w420:dbl)
          n211 = Subtract(x=w421, y=w419) -> (x-y=w428:dbl)
          n212 = Subtract(x=w420, y=w419) -> (x-y=w427:dbl)
          n213 = Bundle(w428, w427) -> (w426:cluster{dbl, dbl})  [unwired: 1 in]
          n214 = call "IMAQ Overlay Line"("Color"=w415, "End Point"=w426, "Start Point"=w422, "Image"=w431) -> ("Image Out"=w430:T1)  [unwired: 6 in, 1 out]
          n215 = Unbundle(w422) -> (w418:dbl, "Position_Y"=w416:dbl)
          n216 = Subtract(x=w418, y=w417) -> (x-y=w424:dbl)
          n217 = Add(x=w416, y=w417) -> (x+y=w425:dbl)
          n218 = Bundle(w424, w425) -> (w423:cluster{dbl, dbl})  [unwired: 1 in]
          n219 = call "IMAQ Overlay Line"("Color"=w415, "End Point"=w423, "Start Point"=w422, "Image"=w430) -> ("Image Out"=w429:T1)  [unwired: 6 in, 1 out]
        }
        frame Enabled {
        }
      }
    }
    frame 7 {
      (unwired) "Caliper"
      n220 = Array Subset(array=w481, length=3) -> (w482:T5[])  [unwired: 1 in]
      n221 = Unbundle By Name(w479) -> ()  [unwired: 1 out]
      n222 = for {
        tunnel: w482 -> [w496] mode=indexing
        tunnel: w480 -> [w494]
        shift-right: [w489] -> w476
        shift-left: w478 -> [w492]
        tunnel: [w484] -> w467
        tunnel: [w485] -> w477 mode=indexing
        tunnel: w466 -> [w484]
        i -> [w488]
        n223 = Unbundle By Name(w496) -> ("Type"=w495:T6, "Index"=w493:i32)
        n224 = Increment(x=w488) -> (x+1=w486:i32)
        n225 = case shown="\"CaliperResult\"" w495 {
          tunnel: w494 -> [w504 _]
          tunnel: w493 -> [w503 _]
          tunnel: [w499 _] -> w485
          tunnel: [FALSE ("StepError?") _] -> _
          tunnel: w492 -> [w497 w505]
          tunnel: [w497 w505] -> w491
          frame "AnalysisResult", Default {
            n226 = Index Array(array=w504, index=w503) -> (element=w502:T2)
            n227 = Unbundle By Name(w502) -> ("Position_X"=w501:dbl, "Position_Y"=w500:dbl)
            n228 = Bundle("Position_X"=w501, "Position_Y"=w500) -> (w499:cluster{"Position_X":dbl, "Position_Y":dbl})  [unwired: 1 in]
          }
          frame "CaliperResult" {
          }
        }
        n229 = Number To Decimal String(number=w486) -> (decimal integer string=w487:string)  [unwired: 1 in]
        n230 = call "Draw Overlay Point.vi"("Color"=w484, "Cluster"=w485, "Refnum in"=w491) -> ("Refnum out"=w490:T1)  [unwired: 8 in]
        n231 = call "IMAQ Overlay Text"("Text Color (black)"=w484, "String"=w487, "Origin"=w485, "Image"=w490) -> ("Image Out"=w489:T1)  [unwired: 6 in, 1 out]
      }
      n232 = Index Array(array=w477, index #1=1 ("index"), index #2=0 ("index"), index #3=2 ("index")) -> (element #1=w470:cluster{"Position_X":dbl, "Position_Y":dbl}, element #2=w471:cluster{"Position_X":dbl, "Position_Y":dbl}, element #3=w469:cluster{"Position_X":dbl, "Position_Y":dbl})
      n233 = call "IMAQ Overlay Line"("Color"=w467, "End Point"=w470, "Start Point"=w471, "Image"=w476) -> ("Image Out"=w474:T1)  [unwired: 6 in, 1 out]
      n234 = call "IMAQ Overlay Line"("Color"=w467, "End Point"=w469, "Start Point"=w470, "Image"=w474) -> ("Image Out"=w468:T1)  [unwired: 6 in, 1 out]
    }
    frame 8 {
      w517 = 2.0 ("y")
      n235 = Unbundle By Name(w538) -> ("Result.Position.X"=w531:dbl, "Result.Position.Y"=w530:dbl, "Result.P2.X"=w529:dbl, "Result.P2.Y"=w528:dbl)
      n236 = Array Subset(array=w540, length=4) -> (w541:T5[])  [unwired: 1 in]
      n237 = for {
        tunnel: w541 -> [w555] mode=indexing
        tunnel: w539 -> [w553]
        shift-right: [w548] -> w535
        shift-left: w537 -> [w551]
        tunnel: [w543] -> w506
        tunnel: [w544] -> w536 mode=indexing
        tunnel: w507 -> [w543]
        i -> [w547]
        n238 = Unbundle By Name(w555) -> ("Type"=w554:T6, "Index"=w552:i32)
        n239 = Increment(x=w547) -> (x+1=w545:i32)
        n240 = case shown="\"CaliperResult\"" w554 {
          tunnel: w553 -> [w563 _]
          tunnel: w552 -> [w562 _]
          tunnel: [w558 _] -> w544
          tunnel: [FALSE ("StepError?") _] -> _
          tunnel: w551 -> [w556 w564]
          tunnel: [w556 w564] -> w550
          frame "AnalysisResult", Default {
            n241 = Index Array(array=w563, index=w562) -> (element=w561:T2)
            n242 = Unbundle By Name(w561) -> ("Position_X"=w560:dbl, "Position_Y"=w559:dbl)
            n243 = Bundle("Position_X"=w560, "Position_Y"=w559) -> (w558:cluster{"Position_X":dbl, "Position_Y":dbl})  [unwired: 1 in]
          }
          frame "CaliperResult" {
          }
        }
        n244 = Number To Decimal String(number=w545) -> (decimal integer string=w546:string)  [unwired: 1 in]
        n245 = call "Draw Overlay Point.vi"("Color"=w543, "Cluster"=w544, "Refnum in"=w550) -> ("Refnum out"=w549:T1)  [unwired: 8 in]
        n246 = call "IMAQ Overlay Text"("Text Color (black)"=w543, "String"=w546, "Origin"=w544, "Image"=w549) -> ("Image Out"=w548:T1)  [unwired: 6 in, 1 out]
      }
      n247 = Bundle("P2.X"=w529, "P2.Y"=w528) -> (w513:cluster{"P2.X":dbl, "P2.Y":dbl})  [unwired: 1 in]
      n248 = Bundle("Position.X"=w531, "Position.Y"=w530) -> (w514:cluster{"Position.X":dbl, "Position.Y":dbl})  [unwired: 1 in]
      n249 = Index Array(array=w536) -> (element #1=w511:cluster{"Position_X":dbl, "Position_Y":dbl}, element #2=w510:cluster{"Position_X":dbl, "Position_Y":dbl}, element #3=w509:cluster{"Position_X":dbl, "Position_Y":dbl}, element #4=w508:cluster{"Position_X":dbl, "Position_Y":dbl})  [unwired: 4 in]
      n250 = call "IMAQ Overlay Line"("Color"=w506, "End Point"=w510, "Start Point"=w511, "Image"=w535) -> ("Image Out"=w534:T1)  [unwired: 6 in, 1 out]
      n251 = call "IMAQ Overlay Line"("Color"=w506, "End Point"=w508, "Start Point"=w509, "Image"=w534) -> ("Image Out"=w533:T1)  [unwired: 6 in, 1 out]
      n252 = call "Draw Overlay Point.vi"("Color"=w506, "Cluster"=w514, "Refnum in"=w533) -> ("Refnum out"=w532:T1)  [unwired: 8 in]
      n253 = call "Draw Overlay Point.vi"("Color"=w506, "Cluster"=w513, "Refnum in"=w532) -> ("Refnum out"=w527:T1)  [unwired: 8 in]
      n254 = Unbundle(w514) -> ("Position.X"=w523:dbl, "Position.Y"=w520:dbl)
      n255 = Unbundle(w513) -> ("P2.X"=w521:dbl, "P2.Y"=w522:dbl)
      n256 = Add(x=w523, y=w521) -> (x+y=w519:dbl)
      n257 = Add(x=w520, y=w522) -> (x+y=w518:dbl)
      n258 = call "IMAQ Overlay Line"("Color"=w506, "End Point"=w513, "Start Point"=w514, "Image"=w527) -> ("Image Out"=w526:T1)  [unwired: 6 in, 1 out]
      n259 = Divide(x=w519, y=w517) -> (x/y=w516:dbl)
      n260 = Divide(x=w518, y=w517) -> (x/y=w515:dbl)
      n261 = Bundle(w516, w515) -> (w512:cluster{dbl, dbl})  [unwired: 1 in]
      n262 = call "IMAQ Overlay Text"("Text Color (black)"=w506, "String"="Caliper", "Origin"=w512, "Image"=w526) -> ("Image Out"=w525:T1)  [unwired: 6 in, 1 out]
    }
    frame 11 {
      w575 = 2.0 ("y")
      n263 = Unbundle By Name(w597) -> ("Result.Position.X"=w590:dbl, "Result.Position.Y"=w589:dbl, "Result.P2.X"=w588:dbl, "Result.P2.Y"=w587:dbl)
      n264 = Array Subset(array=w599, length=4) -> (w600:T5[])  [unwired: 1 in]
      n265 = for {
        tunnel: w600 -> [w614] mode=indexing
        tunnel: w598 -> [w612]
        shift-right: [w607] -> w594
        shift-left: w596 -> [w610]
        tunnel: [w602] -> w583
        tunnel: [w603] -> w595 mode=indexing
        tunnel: w565 -> [w602]
        i -> [w606]
        n266 = Unbundle By Name(w614) -> ("Type"=w613:T6, "Index"=w611:i32)
        n267 = Increment(x=w606) -> (x+1=w604:i32)
        n268 = case shown="\"CaliperResult\"" w613 {
          tunnel: w612 -> [w622 _]
          tunnel: w611 -> [w621 _]
          tunnel: [w617 _] -> w603
          tunnel: [FALSE ("StepError?") _] -> _
          tunnel: w610 -> [w615 w623]
          tunnel: [w615 w623] -> w609
          frame "AnalysisResult", Default {
            n269 = Index Array(array=w622, index=w621) -> (element=w620:T2)
            n270 = Unbundle By Name(w620) -> ("Position_X"=w619:dbl, "Position_Y"=w618:dbl)
            n271 = Bundle("Position_X"=w619, "Position_Y"=w618) -> (w617:cluster{"Position_X":dbl, "Position_Y":dbl})  [unwired: 1 in]
          }
          frame "CaliperResult" {
          }
        }
        n272 = Number To Decimal String(number=w604) -> (decimal integer string=w605:string)  [unwired: 1 in]
        n273 = call "Draw Overlay Point.vi"("Color"=w602, "Cluster"=w603, "Refnum in"=w609) -> ("Refnum out"=w608:T1)  [unwired: 8 in]
        n274 = call "IMAQ Overlay Text"("Text Color (black)"=w602, "String"=w605, "Origin"=w603, "Image"=w608) -> ("Image Out"=w607:T1)  [unwired: 6 in, 1 out]
      }
      n275 = Bundle("P2.X"=w588, "P2.Y"=w587) -> (w571:cluster{"P2.X":dbl, "P2.Y":dbl})  [unwired: 1 in]
      n276 = Bundle("Position.X"=w590, "Position.Y"=w589) -> (w572:cluster{"Position.X":dbl, "Position.Y":dbl})  [unwired: 1 in]
      n277 = Index Array(array=w595) -> (element #1=w569:cluster{"Position_X":dbl, "Position_Y":dbl}, element #2=w568:cluster{"Position_X":dbl, "Position_Y":dbl}, element #3=w567:cluster{"Position_X":dbl, "Position_Y":dbl}, element #4=w566:cluster{"Position_X":dbl, "Position_Y":dbl})  [unwired: 4 in]
      n278 = call "IMAQ Overlay Line"("Color"=w583, "End Point"=w568, "Start Point"=w569, "Image"=w594) -> ("Image Out"=w593:T1)  [unwired: 6 in, 1 out]
      n279 = call "IMAQ Overlay Line"("Color"=w583, "End Point"=w566, "Start Point"=w567, "Image"=w593) -> ("Image Out"=w592:T1)  [unwired: 6 in, 1 out]
      n280 = call "Draw Overlay Point.vi"("Color"=w583, "Cluster"=w572, "Refnum in"=w592) -> ("Refnum out"=w591:T1)  [unwired: 8 in]
      n281 = call "Draw Overlay Point.vi"("Color"=w583, "Cluster"=w571, "Refnum in"=w591) -> ("Refnum out"=w586:T1)  [unwired: 8 in]
      n282 = Unbundle(w572) -> ("Position.X"=w581:dbl, "Position.Y"=w578:dbl)
      n283 = Unbundle(w571) -> ("P2.X"=w579:dbl, "P2.Y"=w580:dbl)
      n284 = Add(x=w581, y=w579) -> (x+y=w577:dbl)
      n285 = Add(x=w578, y=w580) -> (x+y=w576:dbl)
      n286 = call "IMAQ Overlay Line"("Color"=w583, "End Point"=w571, "Start Point"=w572, "Image"=w586) -> ("Image Out"=w585:T1)  [unwired: 6 in, 1 out]
      n287 = Divide(x=w577, y=w575) -> (x/y=w574:dbl)
      n288 = Divide(x=w576, y=w575) -> (x/y=w573:dbl)
      n289 = Bundle(w574, w573) -> (w570:cluster{dbl, dbl})  [unwired: 1 in]
      n290 = call "IMAQ Overlay Text"("Text Color (black)"=w583, "String"="Caliper", "Origin"=w570, "Image"=w585) -> ("Image Out"=w584:T1)  [unwired: 6 in, 1 out]
    }
    frame 9 {
      w633 = 2.0 ("y")
      # "輸出中線"
      # "Mid Line尋找點與線中間的中線"
      n291 = Unbundle By Name(w653) -> ("Result.Position.X"=w648:dbl, "Result.Position.Y"=w647:dbl, "Result.P2.X"=w646:dbl, "Result.P2.Y"=w645:dbl)
      n292 = Array Subset(array=w655, length=4) -> (w656:T5[])  [unwired: 1 in]
      n293 = for {
        tunnel: w656 -> [w670] mode=indexing
        tunnel: w654 -> [w668]
        shift-right: [w663] -> w650
        shift-left: w652 -> [w666]
        tunnel: [w658] -> w641
        tunnel: [w659] -> w651 mode=indexing
        tunnel: w624 -> [w658]
        i -> [w662]
        # "輸入第一點與第二點為直線第三點為中點"
        n294 = Unbundle By Name(w670) -> ("Type"=w669:T6, "Index"=w667:i32)
        n295 = Increment(x=w662) -> (x+1=w660:i32)
        n296 = case shown="\"CaliperResult\"" w669 {
          tunnel: w668 -> [w678 _]
          tunnel: w667 -> [w677 _]
          tunnel: [w673 _] -> w659
          tunnel: [FALSE ("StepError?") _] -> _
          tunnel: w666 -> [w671 w679]
          tunnel: [w671 w679] -> w665
          frame "AnalysisResult", Default {
            n297 = Index Array(array=w678, index=w677) -> (element=w676:T2)
            n298 = Unbundle By Name(w676) -> ("Position_X"=w675:dbl, "Position_Y"=w674:dbl)
            n299 = Bundle("Position_X"=w675, "Position_Y"=w674) -> (w673:cluster{"Position_X":dbl, "Position_Y":dbl})  [unwired: 1 in]
          }
          frame "CaliperResult" {
          }
        }
        n300 = Number To Decimal String(number=w660) -> (decimal integer string=w661:string)  [unwired: 1 in]
        n301 = call "Draw Overlay Point.vi"("Color"=w658, "Cluster"=w659, "Refnum in"=w665) -> ("Refnum out"=w664:T1)  [unwired: 8 in]
        n302 = call "IMAQ Overlay Text"("Text Color (black)"=w658, "String"=w661, "Origin"=w659, "Image"=w664) -> ("Image Out"=w663:T1)  [unwired: 6 in, 1 out]
      }
      n303 = Bundle("P2.X"=w646, "P2.Y"=w645) -> (w629:cluster{"P2.X":dbl, "P2.Y":dbl})  [unwired: 1 in]
      n304 = Bundle("Position.X"=w648, "Position.Y"=w647) -> (w630:cluster{"Position.X":dbl, "Position.Y":dbl})  [unwired: 1 in]
      n305 = Index Array(array=w651) -> (element #1=w627:cluster{"Position_X":dbl, "Position_Y":dbl}, element #2=w626:cluster{"Position_X":dbl, "Position_Y":dbl})  [unwired: 2 in]
      n306 = call "IMAQ Overlay Line"("Color"=w641, "End Point"=w626, "Start Point"=w627, "Image"=w650) -> ("Image Out"=w625:T1)  [unwired: 6 in, 1 out]
      n307 = call "Draw Overlay Point.vi"("Color"=w641, "Cluster"=w630, "Refnum in"=w625) -> ("Refnum out"=w649:T1)  [unwired: 8 in]
      n308 = call "Draw Overlay Point.vi"("Color"=w641, "Cluster"=w629, "Refnum in"=w649) -> ("Refnum out"=w644:T1)  [unwired: 8 in]
      n309 = Unbundle(w630) -> ("Position.X"=w639:dbl, "Position.Y"=w636:dbl)
      n310 = Unbundle(w629) -> ("P2.X"=w637:dbl, "P2.Y"=w638:dbl)
      n311 = Add(x=w639, y=w637) -> (x+y=w635:dbl)
      n312 = Add(x=w636, y=w638) -> (x+y=w634:dbl)
      n313 = call "IMAQ Overlay Line"("Color"=w641, "End Point"=w629, "Start Point"=w630, "Image"=w644) -> ("Image Out"=w643:T1)  [unwired: 6 in, 1 out]
      n314 = Divide(x=w635, y=w633) -> (x/y=w632:dbl)
      n315 = Divide(x=w634, y=w633) -> (x/y=w631:dbl)
      n316 = Bundle(w632, w631) -> (w628:cluster{dbl, dbl})  [unwired: 1 in]
      n317 = call "IMAQ Overlay Text"("Text Color (black)"=w641, "String"="Caliper", "Origin"=w628, "Image"=w643) -> ("Image Out"=w642:T1)  [unwired: 6 in, 1 out]
    }
  }
  "DLL Vision_Image Out" <- w2
